vi "2DWB_to_2DWB_PosNeg_sub.vi"(3 "2DWB_Input":i32[][](array[numeric])=[[-807, -4892, -429, 1215, -1226, -47, -3205, 2911, 17, 733], [-807, -4892, -429, 1215, -1226, -47, -3205, 2911, 17, 733], [-807, -4892, -429, 1215, -1226, -47, -3205, 2911, 17, 733], [-807, -4892, -429, 1215, -1226, -47, -3205, 2911, 17, 733]]) -> (0 "2DWB_OutputNeg":i32[][](array[numeric]), 1 "2DWB_OutputPos":i32[][](array[numeric]))   [LabVIEW 2021]
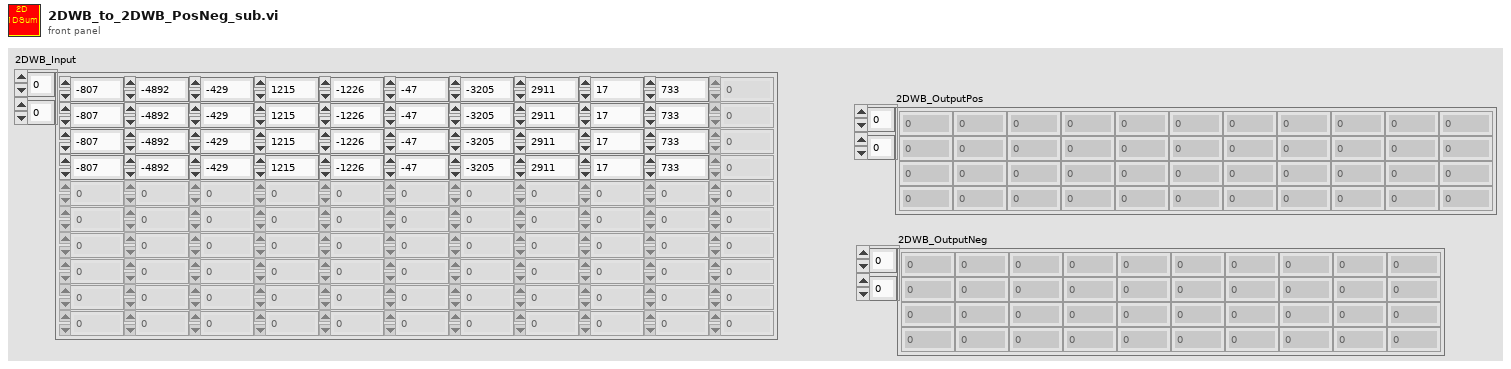
[diagram p1: front panel]
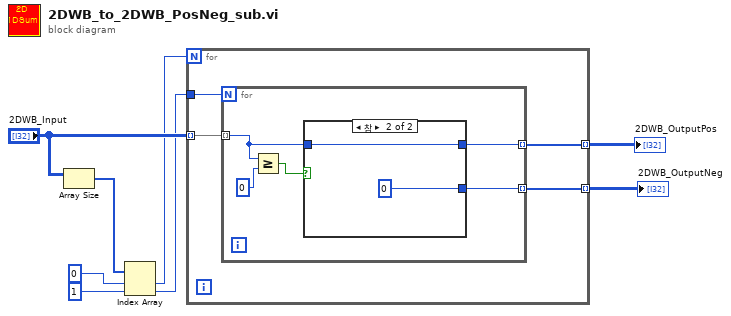
[diagram p0: block diagram]
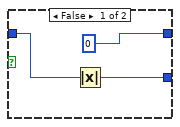
[diagram p2: hidden frame]
diagram:
  n1 = Array Size(array="2DWB_Input") -> (size(s)=w8:i32[])
  n2 = Index Array(array=w8, index #1=0 ("인덱스"), index #2=1 ("인덱스")) -> (element #1=w4:i32, element #2=w3:i32)
  n3 = for {
    N: w4 -> [_]
    tunnel: "2DWB_Input" -> [w11] mode=indexing
    tunnel: w3 -> [w12]
    tunnel: [w10] -> w2 mode=indexing
    tunnel: [w9] -> w1 mode=indexing
    n4 = for {
      N: w12 -> [_]
      tunnel: w11 -> [w15] mode=indexing
      tunnel: [w14] -> w10 mode=indexing
      tunnel: [w13] -> w9 mode=indexing
      n5 = Greater Or Equal?(x=w15, y=0) -> (x >= y?=w17:bool)
      n6 = case shown="참" w17 {
        tunnel: [0 ("y") w22] -> w14
        tunnel: w15 -> [w19 w22]
        tunnel: [w18 0 ("y")] -> w13
        frame False {
          n7 = Absolute Value(x=w19) -> (abs(x)=w18:i32)
        }
        frame True {
        }
      }
    }
  }
  "2DWB_OutputPos" <- w2
  "2DWB_OutputNeg" <- w1
